vi "macro_Pose3d_XYZ_RollPitchYaw_Rad.vi"   [LabVIEW 2019, in "Trajectory_Library.lvlib"]
uses:
  Trajectory_Library.lvlib
types:
  T1 = typedef "Trajectory_Library.lvlib/ROTATION3D.ctl" = cluster{"Q_quaternion":T2}
  T2 = typedef "Trajectory_Library.lvlib/QUATERNION.ctl" = cluster{"R":dbl, "V":dbl[]}
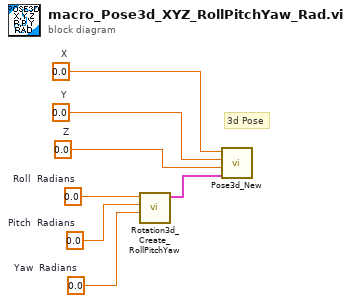
[diagram p0: block diagram]
diagram:
  w3 = 0.0  # X
  w1 = 0.0  # Y
  w4 = 0.0  # Z
  w5 = 0.0  # Roll  Radians
  w6 = 0.0  # Pitch  Radians
  w7 = 0.0  # Yaw  Radians
  # "3d Pose"
  n1 = call "Rotation3d_Create_RollPitchYaw.vi"("Yaw"=w7, "Pitch"=w6, "Roll"=w5) -> ("Rotation3d"=w2:T1)  [unwired: 8 in]
  n2 = call "Pose3d_New.vi"("Rotation3d"=w2, "z"=w4, "Y"=w1, "X"=w3) -> ()  [unwired: 7 in, 1 out]
